vi "pic_Scale.vi"(8 "error in (no error)":errorcluster, 11 "Graph_ref_in":refnum<vi>) -> (0 "error out":errorcluster, 3 "reference out":refnum<vi>)   [LabVIEW 2020, in "GraphBG_manage.lvlib" / "Graph.lvclass"]
uses:
  Graph.lvclass
  T50/subVI/xyY_graph.ctl
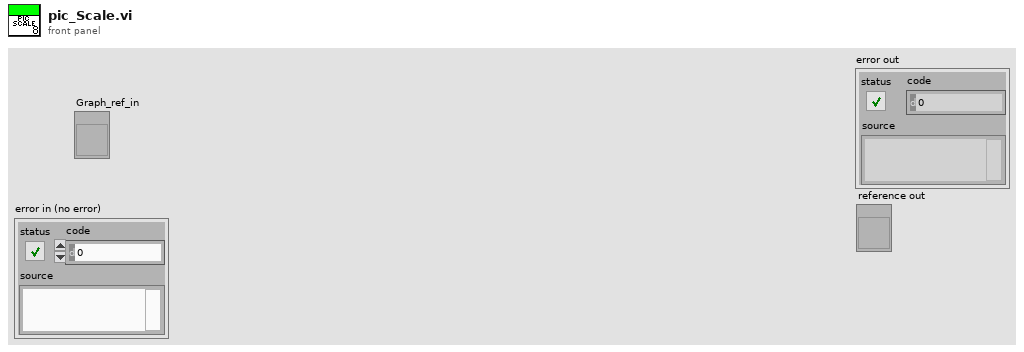
[diagram p1: front panel]
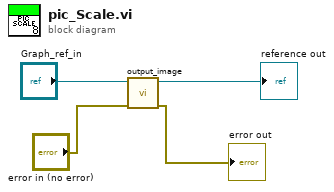
[diagram p0: block diagram]
diagram:
  n1 = call "output_image.vi"("error in (no error)"="error in (no error)", "Graph_ref_in"="Graph_ref_in") -> ("error out"=→"error out":errorcluster, "reference out"=→"reference out":refnum<vi>)  [unwired: 8 in]
